vi "Untitled 1.vi"() -> ()   [LabVIEW 2015, in "SQLite.lvclass"]
uses:
  SQLite.lvclass
  TabelFullName.ctl
  SQLiteFileName.ctl
panel:
  in  "Value 2":string
  in  "stop":bool
  out "Value":string
  out "error out":errorcluster
  out "ColunmsList":string[](array[string])
  out "number (0 to 1)":dbl
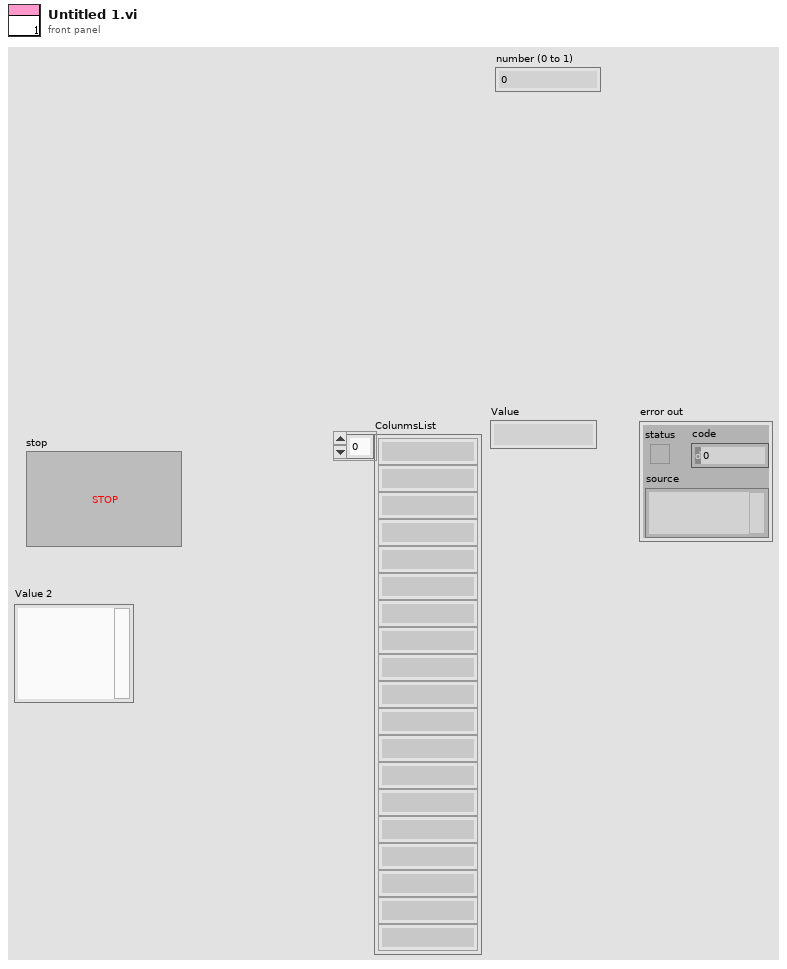
[diagram p1: front panel]
types:
  T1 = typedef "SQLite.lvclass/SQLiteFileName.ctl" = string
  T2 = typedef "SQLite.lvclass/TabelFullName.ctl" = string
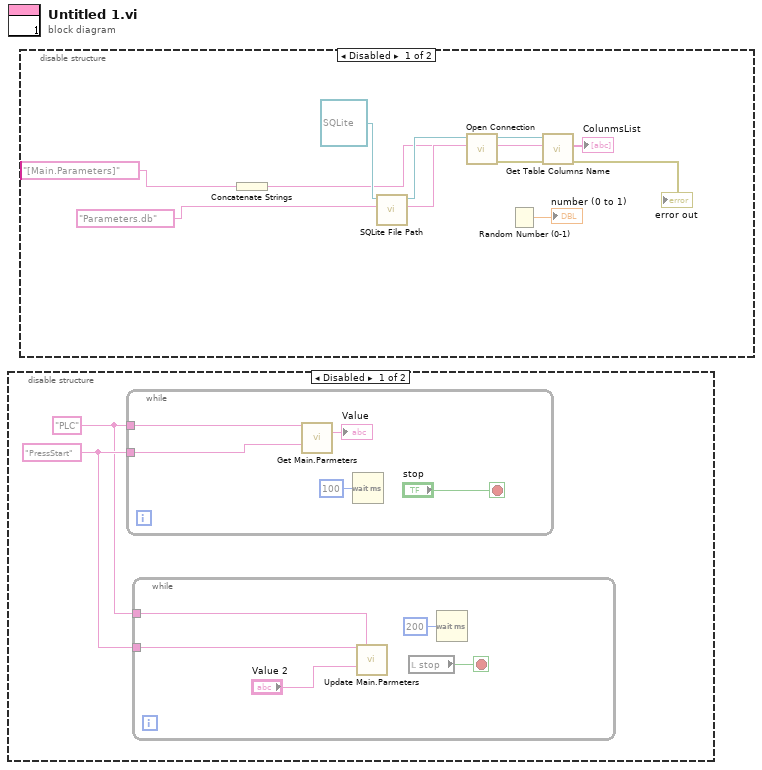
[diagram p0: block diagram]
diagram:
  n1 = disable-structure shown="Disabled" {
    frame Disabled {
      w2 = "PressStart" ("VariableName")
      w1 = "PLC" ("Main")
      n2 = while {
        tunnel: w1 -> [w9]
        tunnel: w2 -> [w8]
        stop <- "stop" stop-if-true
        n3 = call "Get Main.Parmeters.vi"("Main"=w9, "VariableName"=w8) -> ("Value"=→"Value":string)  [unwired: 7 in, 6 out]
        n4 = Wait (ms)(milliseconds to wait=u32 100) -> ()  [unwired: 1 out]
      }
      n5 = while {
        tunnel: w2 -> [w6]
        tunnel: w1 -> [w5]
        stop <- w7 stop-if-true
        n6 = call "Update Main.Parmeters.vi"("VariableName"=w6, "Main"=w5, "Value"="Value 2") -> ()  [unwired: 12 in, 1 out]
        n7 = local read "stop"() -> (w7:bool)
        n8 = Wait (ms)(milliseconds to wait=u32 200) -> ()  [unwired: 1 out]
      }
    }
    frame Enabled {
    }
  }
  n9 = disable-structure shown="Disabled" {
    frame Disabled {
      n10 = Concatenate Strings(T2 "[Main.Parameters]" ("TabelFullName")) -> (w18:string)
      n11 = call "SQLite File Path.vi"("SQLiteFileName"=T1 "Parameters.db", "SQLite in"=refnum<class "SQLite.lvclass"> refnum ("SQLite.lvclass")) -> ("string"=w20:string, "SQLite out"=w22:refnum<class "SQLite.lvclass">)  [unwired: 7 in, 1 out]
      n12 = call-dynamic "Open Connection.vi"("ConnectionString"=w20, "HostDB in"=w22) -> ("error out"=w19:errorcluster, "HostDB out"=w17:refnum<class "SQLite.lvclass">)  [unwired: 8 in]
      n13 = Random Number (0-1)() -> (number: 0 to 1=→"number (0 to 1)":dbl)
      n14 = call-dynamic "Get Table Columns Name.vi"("error in (no error)"=w19, "TableName"=w18, "HostDB in"=w17) -> ("error out"=→"error out":errorcluster, "ColunmsList"=→"ColunmsList":string[])  [unwired: 4 in, 3 out]
    }
    frame Enabled {
    }
  }
